vi "Find SLSC Switch Custom Device by Slot Number.vi"(8 "error in (no error)":errorcluster, 10 "slot number":u32, 11 "Target in":refnum<k24>) -> (0 "error out":errorcluster, 2 "SLSC Switch Custom Device Ref":T1=18446744073709551615 format="%.0x", 3 "Target out":refnum<k24>)   [LabVIEW 2017, in "SLSC Switch Scripting.lvlib"]
uses:
  SLSC Switch Scripting.lvlib
  NationalInstruments.VeriStand.SystemDefinitionAPI
  <vilib>/NI Veristand/Custom Device API/Custom Device Item Ref.ctl
  Shared/Constants.vi
  Shared/SLSC Switch Shared.lvlib
  <vilib>/NI Veristand/Custom Device API/Custom Device API.lvlib
panel:
  in  "error message":string="The item at the specified slot number is not an SLSC Switch custom device."
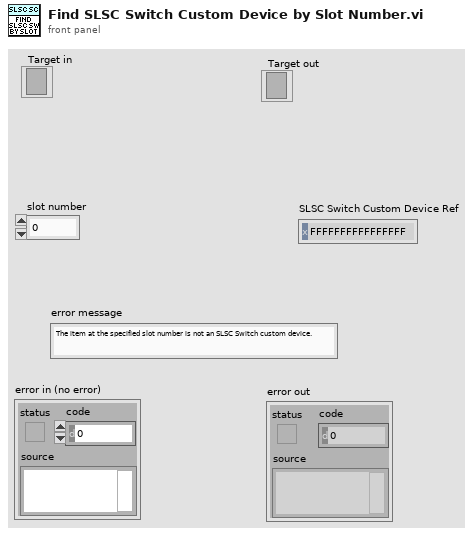
[diagram p1: front panel]
types:
  T1 = typedef "Custom Device API.lvlib/Custom Device Item Ref.ctl" = u64
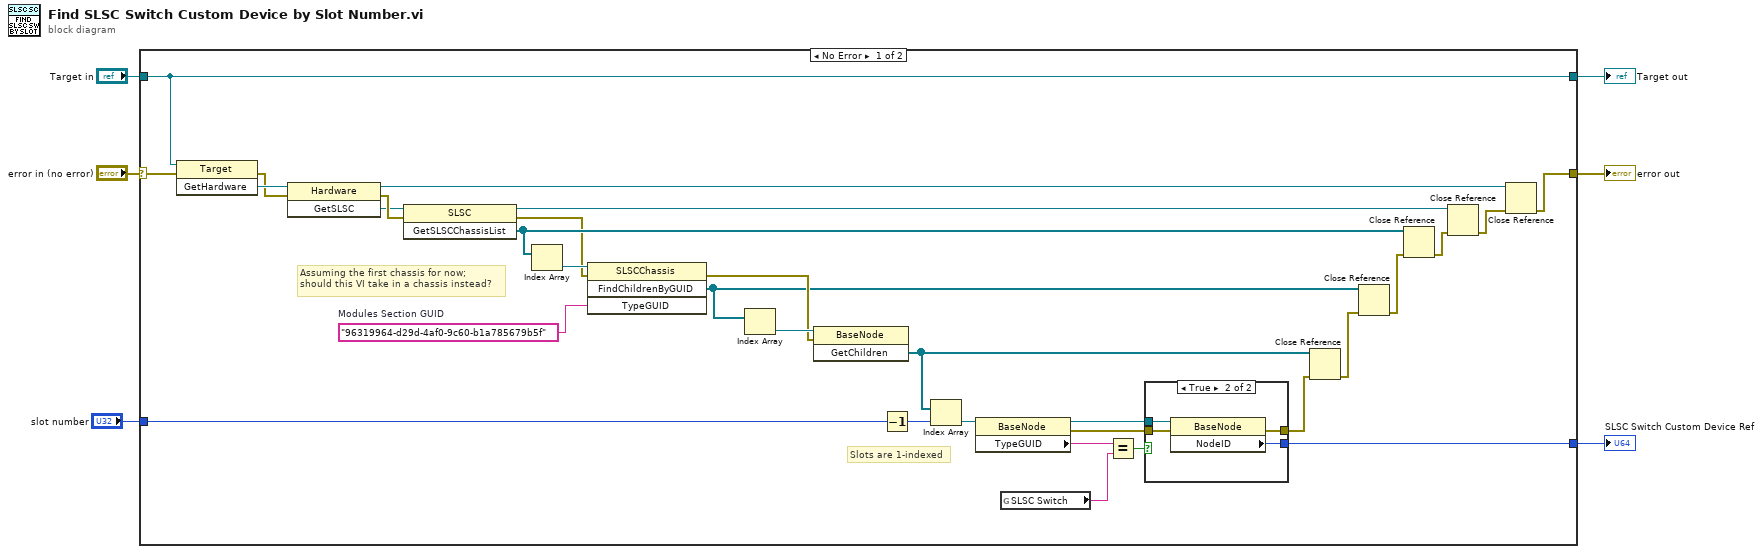
[diagram p0: block diagram]
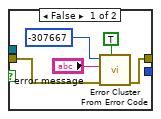
[diagram p2: hidden frame]
diagram:
  n1 = case shown="No Error" "error in (no error)" {
    selector: "error in (no error)" -> [w28 w48]
    tunnel: [w22 w48] -> w3
    tunnel: "Target in" -> [w25 w47]
    tunnel: [w25 w47] -> w4
    tunnel: "slot number" -> [w36 _]
    tunnel: [w31 _] -> w1
    frame No Error {
      w14 = "96319964-d29d-4af0-9c60-b1a785679b5f"  # Modules Section GUID
      # "Assuming the first chassis for now;\nshould this VI take in a chassis instead?"
      # "Slots are 1-indexed"
      n2 = invoke class="Target" method="GetHardware"(reference=w25, error in=w28) -> (error out=w24:errorcluster, "GetHardware"=w29:refnum<k24>)  [unwired: 1 in, 1 out]
      n3 = invoke class="Hardware" method="GetSLSC"(reference=w29, error in=w24) -> (reference out=w23:refnum<k24>, error out=w27:errorcluster, "GetSLSC"=w26:refnum<k24>)  [unwired: 1 in]
      n4 = invoke class="SLSC" method="GetSLSCChassisList"(reference=w26, error in=w27) -> (reference out=w21:refnum<k24>, error out=w11:errorcluster, "GetSLSCChassisList"=w18:refnum<k24>[])  [unwired: 1 in]
      n5 = Index Array(array=w18) -> (element=w13:refnum<k24>)  [unwired: 1 in]
      n6 = invoke class="SLSCChassis" method="FindChildrenByGUID"(reference=w13, error in=w11, "TypeGUID"=w14) -> (error out=w10:errorcluster, "FindChildrenByGUID"=w7:refnum<k24>[])  [unwired: 1 in, 2 out]
      n7 = Index Array(array=w7) -> (element=w12:refnum<k24>)  [unwired: 1 in]
      n8 = invoke class="BaseNode" method="GetChildren"(reference=w12, error in=w10) -> ("GetChildren"=w16:refnum<k24>[])  [unwired: 1 in, 2 out]
      n9 = Decrement(x=w36) -> (x-1=w37:u32)
      n10 = Index Array(array=w16, index=w37) -> (element=w17:refnum<k24>)
      n11 = property class="BaseNode"(reference=w17) -> (reference out=w30:refnum<k24>, error out=w33:errorcluster, "TypeGUID"=w35:string)  [unwired: 1 in]
      n12 = global read "Constants.vi" "SLSC Switch"() -> (w34:string)
      n13 = Equal?(x=w35, y=w34) -> (x = y?=w32:bool)
      n14 = case shown="True" w32 {
        tunnel: w33 -> [w41 w46]
        tunnel: [_ w45] -> w31
        tunnel: [w42 w44] -> w15
        tunnel: w30 -> [_ w43]
        frame False {
          n15 = call <vilib>:"Error Cluster From Error Code.vi"("show call chain? (False)"=TRUE, "error in (no error)"=w41, "error message (\"\")"="error message", "error code (0)"=-307667) -> ("error out"=w42:errorcluster)  [unwired: 5 in]
        }
        frame True {
          n16 = property class="BaseNode"(reference=w43, error in=w46) -> (error out=w44:errorcluster, "NodeID"=w45:u64)  [unwired: 1 out]
        }
      }
      n17 = Close Reference(reference=w16, error in (no error)=w15) -> (error out=w9:errorcluster)
      n18 = Close Reference(reference=w7, error in (no error)=w9) -> (error out=w8:errorcluster)
      n19 = Close Reference(reference=w18, error in (no error)=w8) -> (error out=w20:errorcluster)
      n20 = Close Reference(reference=w21, error in (no error)=w20) -> (error out=w19:errorcluster)
      n21 = Close Reference(reference=w23, error in (no error)=w19) -> (error out=w22:errorcluster)
    }
    frame Error {
    }
  }
  "Target out" <- w4
  "error out" <- w3
  "SLSC Switch Custom Device Ref" <- w1
